vi "Get associated LV error.vi"(11 "ErrorHandler JSON in":refnum<class "ErrorHandler JSON.lvclass">) -> (2 "Associated LabVIEW Error":errorcluster, 3 "ErrorHandler JSON out":refnum<class "ErrorHandler JSON.lvclass">)   [LabVIEW 2020, in "wamplv.lvlib" / "ErrorHandler JSON.lvclass"]
uses:
  ErrorHandler JSON.lvclass
  ErrorHandler JSON.lvclass/ErrorHandler JSON.ctl
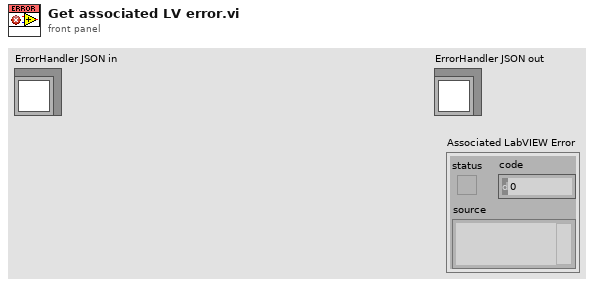
[diagram p1: front panel]
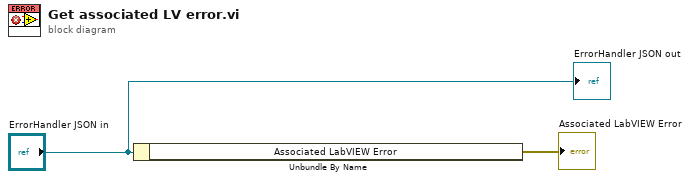
[diagram p0: block diagram]
diagram:
  n1 = Unbundle By Name("ErrorHandler JSON in") -> ("Associated LabVIEW Error"=→"Associated LabVIEW Error":errorcluster)
  "ErrorHandler JSON out" <- "ErrorHandler JSON in"
